vi "ManageShortcutMenu.vi"(9 "Run Mode?":bool, 10 "Display State In":T1 caption="State", 11 "MenuRef":refnum<k9>) -> ()   [LabVIEW 2013, in "VariantXControl__VP.xctl"]
uses:
  VariantXControl__VP.xctl
  VariantState.ctl
  Permissions.ctl
  TreeSettings.ctl
  <userlib>/_OpenG.lib/array/array.llb/Conditional Auto-Indexing Tunnel (Variant)__ogtk.vi
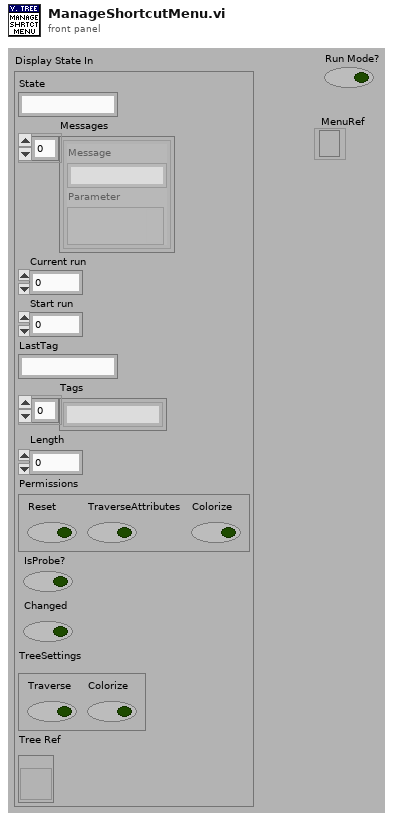
[diagram p1: front panel]
types:
  T1 = typedef "VariantXControl__VP.xctl/VariantState.ctl" = cluster{"State":string, "Messages":cluster{"Message":string, "Parameter":variant}[], "Current run":i32, "Start run":i32, "LastTag":string, "Tags":string[], "Length":i32, "Permissions":T2, "IsProbe?":bool, "Changed":bool, "TreeSettings":T3, "Tree Ref":refnum<vi>}
  T2 = typedef "VariantXControl__VP.xctl/Permissions.ctl" = cluster{"Reset":bool, "TraverseAttributes":bool, "Colorize":bool}
  T3 = typedef "VariantXControl__VP.xctl/TreeSettings.ctl" = cluster{"Traverse":bool, "Colorize":bool}
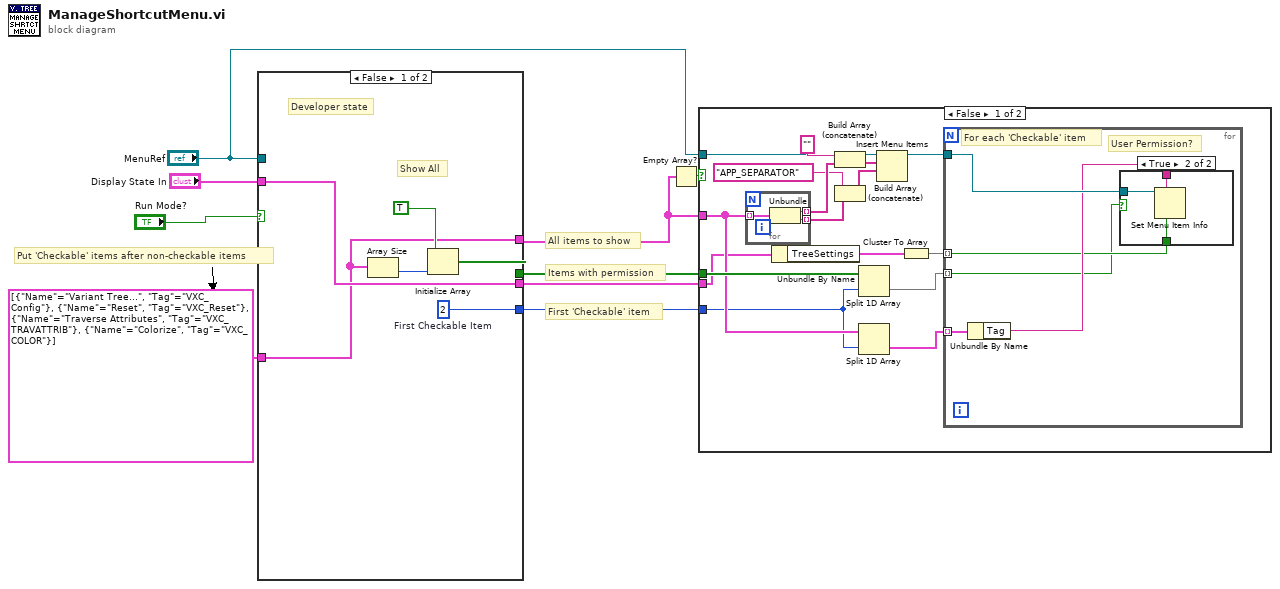
[diagram p0: block diagram]
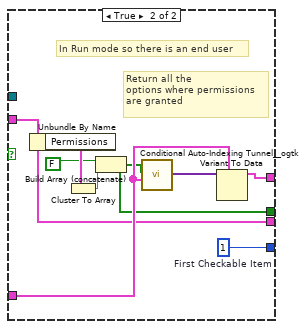
[diagram p4: hidden frame]
diagram:
  # "Items with permission"
  # "First 'Checkable' item"
  # "All items to show"
  # "Put 'Checkable' items after non-checkable items"
  n1 = case shown="False" "Run Mode?" {
    tunnel: "MenuRef" -> [_ _]
    tunnel: "Display State In" -> [w15 w20]
    tunnel: cluster{"Name":string, "Tag":string}[] [{"Name"="Variant Tree...", "Tag"="VXC_Config"}, {"Name"="Reset", "Tag"="VXC_Reset"}, {"Name"="Traverse Attributes", "Tag"="VXC_TRAVATTRIB"}, {"Name"="Colorize", "Tag"="VXC_COLOR"}] -> [w10 w22]
    tunnel: [w10 w21] -> w5
    tunnel: [w12 w16] -> w3
    tunnel: [w15 w20] -> w2
    tunnel: [w14 w19] -> w1
    frame False {
      w14 = 2  # First Checkable Item
      # "Developer state"
      # "Show All"
      n2 = Array Size(array=w10) -> (size(s)=w13:i32)
      n3 = Initialize Array(TRUE, w13) -> (w12:bool[])
    }
    frame True {
      w19 = 1  # First Checkable Item
      # "In Run mode so there is an end user"
      # "Return all the \noptions where permissions\nare granted"
      n4 = Unbundle By Name(w20) -> ("Permissions"=w24:T2)
      n5 = Cluster To Array(cluster=w24) -> (array=w17:bool[])
      n6 = Build Array (concatenate)(FALSE, w17) -> (w16:bool[])
      n7 = call-poly <userlib>:"Conditional Auto-Indexing Tunnel__ogtk.vi"("Array in"=w22, "Elements to keep"=w16) -> ("Filtered Array out"=w23:variant[])  [unwired: 5 in]
      n8 = Variant To Data(type=w22, Variant=w23) -> (data=w21:cluster{"Name":string, "Tag":string}[])  [unwired: 1 in, 1 out]
    }
  }
  n9 = Empty Array?(array=w5) -> (empty?=w6:bool)
  n10 = case shown="False" w6 {
    tunnel: w5 -> [w32 _]
    tunnel: w3 -> [w33 _]
    tunnel: w2 -> [w31 _]
    tunnel: "MenuRef" -> [w28 _]
    tunnel: w1 -> [w27 _]
    frame False {
      n11 = for {
        tunnel: w32 -> [w51] mode=indexing
        tunnel: [w50] -> w40 mode=indexing
        tunnel: [w49] -> w36 mode=indexing
        n12 = Unbundle(w51) -> ("Name"=w50:string, "Tag"=w49:string)
      }
      n13 = Unbundle By Name(w31) -> ("TreeSettings"=w29:T3)
      n14 = Build Array (concatenate)("", w40) -> (w38:string[])
      n15 = Build Array (concatenate)("APP_SEPARATOR", w36) -> (w37:string[])
      n16 = Split 1D Array(array=w33, index=w27) -> (second subarray=w26:bool[])  [unwired: 1 out]
      n17 = Split 1D Array(array=w32, index=w27) -> (second subarray=w25:cluster{"Name":string, "Tag":string}[])  [unwired: 1 out]
      n18 = Insert Menu Items(7:w37, 8:w38, 9:w28) -> (3:w34:refnum<k9>)  [unwired: 3 in, 2 out]
      n19 = Cluster To Array(cluster=w29) -> (array=w30:bool[])
      n20 = for {
        tunnel: w34 -> [w45]
        tunnel: w30 -> [w42] mode=indexing
        tunnel: w26 -> [w41] mode=indexing
        tunnel: w25 -> [w44] mode=indexing
        # "User Permission?"
        # "For each 'Checkable' item"
        n21 = Unbundle By Name(w44) -> ("Tag"=w43:string)
        n22 = case shown="True" w41 {
          tunnel: w45 -> [_ w48]
          tunnel: w43 -> [_ w47]
          tunnel: w42 -> [_ w46]
          frame False {
          }
          frame True {
            n23 = Set Menu Item Info(6:w46, 7:w47, 11:w48) -> ()  [unwired: 4 in, 2 out]
          }
        }
      }
    }
    frame True {
    }
  }
